vi "TAMAÑO.vi"(8 "DISPLONG 3":i32, 9 "DISPLONG 2":i32, 10 "DISPLONG 1":i32) -> (2 "result":i32)   [LabVIEW 2016]
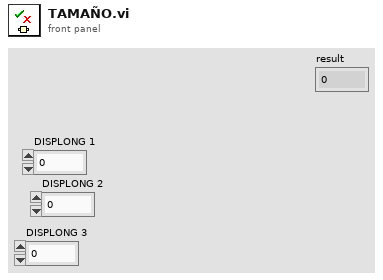
[diagram p1: front panel]
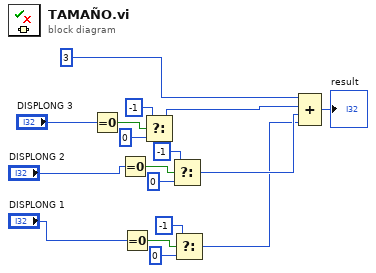
[diagram p0: block diagram]
diagram:
  n1 = Equal To 0?(x="DISPLONG 3") -> (x = 0?=w15:bool)
  n2 = Equal To 0?(x="DISPLONG 2") -> (x = 0?=w12:bool)
  n3 = Equal To 0?(x="DISPLONG 1") -> (x = 0?=w9:bool)
  n4 = Select(t=-1, s=w15, f=0) -> (s? t:f=w4:i32)
  n5 = Select(t=-1, s=w12, f=0) -> (s? t:f=w3:i32)
  n6 = Select(t=-1, s=w9, f=0) -> (s? t:f=w2:i32)
  n7 = Compound Arithmetic op=ADD(3, w4, w3, w2) -> (→"result":i32)
